vi "Actor Core.vi"(8 "error in":errorcluster, 11 "Vision in":refnum<class "Vision.lvclass">) -> (0 "error out":errorcluster, 3 "Actor out":refnum<class "Actor.lvclass">)   [LabVIEW 2022 SP3, in "Vision.lvlib" / "Vision.lvclass"]
doc: "(<B>Filename</B>: Actor Framework.lvlib:Actor.lvclass:Actor Core.vi)\n\nReceives messages to the actor, reacts to them, and initiates any error handling that may shut the actor down.\n\nDescendant classes may override this VI to append parallel tasks for the actor to complete while it handles messages. Overrides use the Call Parent Class Method node."
uses:
  Vision.lvclass
  C:/Program Files (x86)/National Instruments/LabVIEW 2022/vi.lib/ActorFramework/Actor/Actor.lvclass
  <vilib>/ActorFramework/Actor/Actor.lvclass
  Vision.lvclass/Vision.ctl
  <vilib>/MGI/Monitored Actor/Monitored Actor/Monitored Actor/Monitored Actor.lvclass
  Vision Receiver/Vision Receiver/Vision Receiver.lvclass
  C:/Program Files (x86)/National Instruments/LabVIEW 2022/vi.lib/MGI/Monitored Actor/Monitored Actor/Monitored Actor/Monitored Actor.lvclass
  C:/Users/ebert/Documents/codes/ssl/repo/Phoenix Reborn/Vision Receiver/Vision Receiver/Vision Receiver.lvclass
  C:/Users/ebert/Documents/codes/ssl/repo/Phoenix Reborn/UDP Data Receiver/UDP Data Receiver/UDP Data Receiver.lvclass
  C:/Users/ebert/Documents/codes/ssl/repo/Phoenix Reborn/Vision/Vision/Vision.lvclass
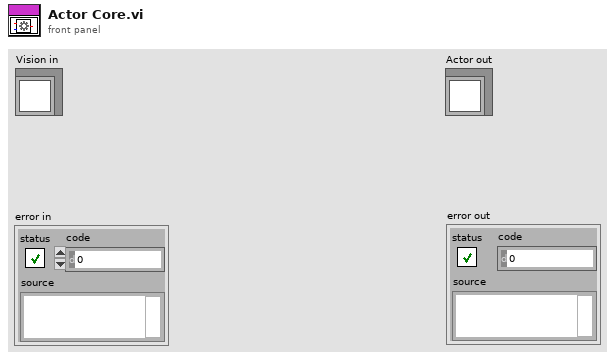
[diagram p1: front panel]
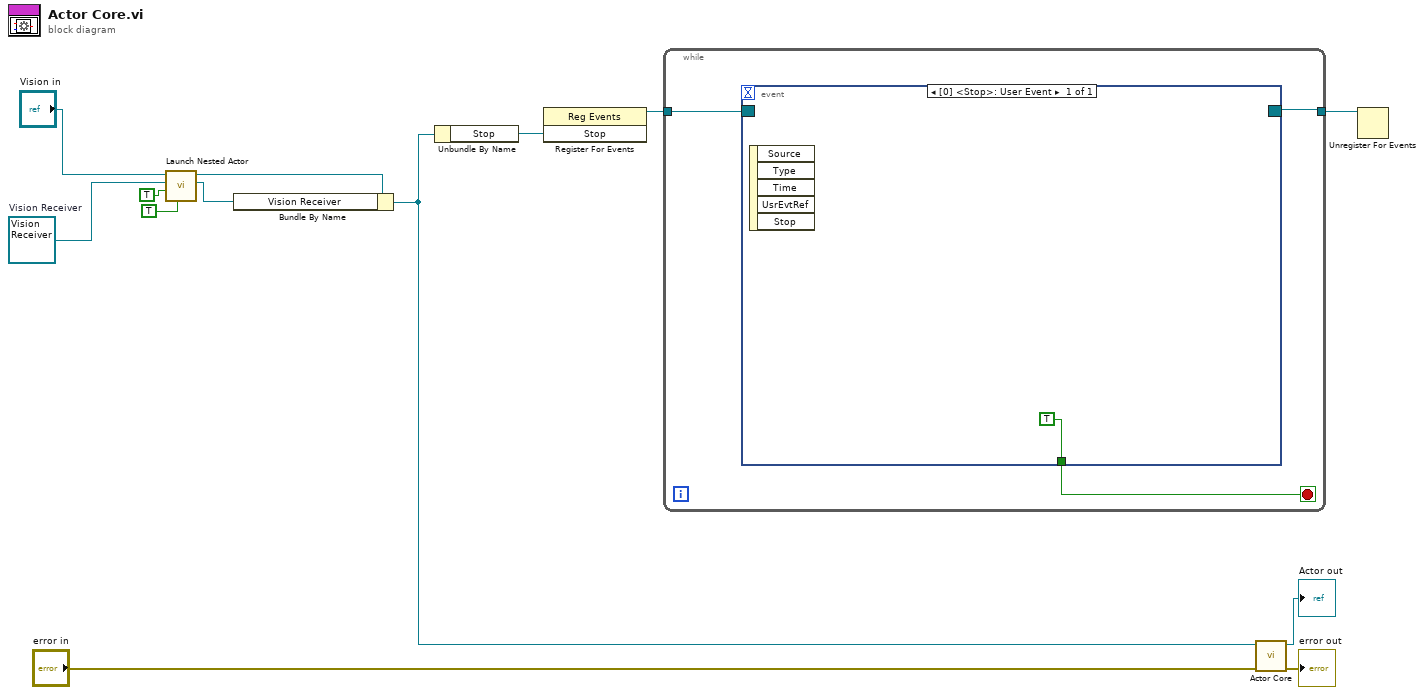
[diagram p0: block diagram]
diagram:
  w1 = refnum<class "Vision Receiver.lvclass"> refnum  # Vision Receiver
  n1 = call <vilib>:"Launch Nested Actor.vi"("Open Actor Core front panel? (F)"=TRUE, "Auto-stop? (T)"=TRUE, "Nested Actor"=w1, "Caller Actor in"="Vision in") -> ("Nested Actor's Enqueuer"=w6:refnum<class "Message Enqueuer.lvclass">, "Caller Actor out"=w5:refnum<class "Vision.lvclass">)  [unwired: 5 in, 1 out]
  n2 = Bundle By Name(cluster=w5, "Vision Receiver"=w6) -> (w3:refnum<class "Vision.lvclass">)
  n3 = Unbundle By Name(w3) -> ("Stop"=w10:refnum<user-event>)
  n4 = register-events(w10) -> (reference out=w9:refnum<event-registration>)  [unwired: 2 in, 1 out]
  n5 = while {
    tunnel: w9 -> [w16]
    tunnel: [w15] -> w8
    stop <- w14 stop-if-true
    n6 = event shown="[0] <Stop>: User Event" {
      selector: w16 -> [_]
      dyn-events: [_] -> w15
      timeout: _ -> [_]
      tunnel: [TRUE] -> w14
      event User Event {
        n7 = event-data() -> ()  [unwired: 1 in, 5 out]
      }
    }
  }
  n8 = call-parent "Actor Core.vi"("error in"="error in", "Actor in"=w3) -> ("error out"=→"error out":errorcluster, "Actor out"=→"Actor out":refnum<class "Actor.lvclass">)  [unwired: 8 in]
  n9 = Unregister For Events(event registration refnum=w8) -> ()  [unwired: 1 in, 1 out]
